vi "MB Serial Receive.vi"(7 "Serial Parameters":T1 {"Slave Address" format="%.0x"}, 8 "error in (no error)":errorcluster, 9 "Timeout":u32=10000, 11 "VISA resource name":refnum<visa-resource-name>) -> (0 "error out":errorcluster, 1 "Exception Code":u8 format="%.0x", 2 "Modbus Data Unit":T2={"Function Code"=1, "Data"=[]} {"Function Code" items=["Read Coils"=1, "Read Discrete Inputs"=2, "Read Holding Registers"=3, "Read Input Registers"=4, "Write Single Coil"=5, "Write Single Register"=6, "Read Exception Status"=7, "Write Multiple Coils"=15, "Write Multiple Registers"=16]; "Data" format="%.0x"}, 3 "VISA resource name out":refnum<visa-resource-name>)   [LabVIEW 2019]
uses:
  MB Modbus Data Unit.ctl
panel:
  out "read modbus frame":errorcluster
  out "read slave address":errorcluster
  # "VI Name: MB Serial Receive.vi\nPurpose: Reads a Modbus message.\nReentrant."
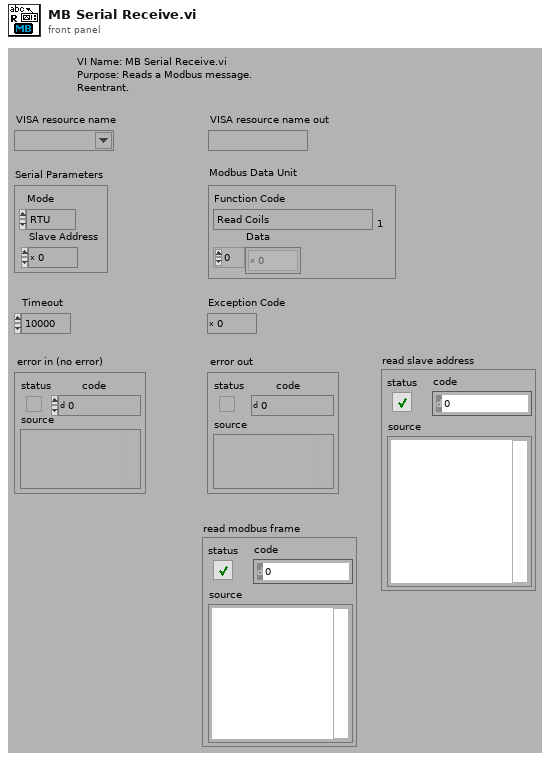
[diagram p1: front panel]
types:
  T1 = cluster{"Mode":enum16{"RTU", "ASCII"}, "Slave Address":u8}
  T2 = typedef "MB Modbus Data Unit.ctl" = cluster{"Function Code":u8, "Data":u8[]}
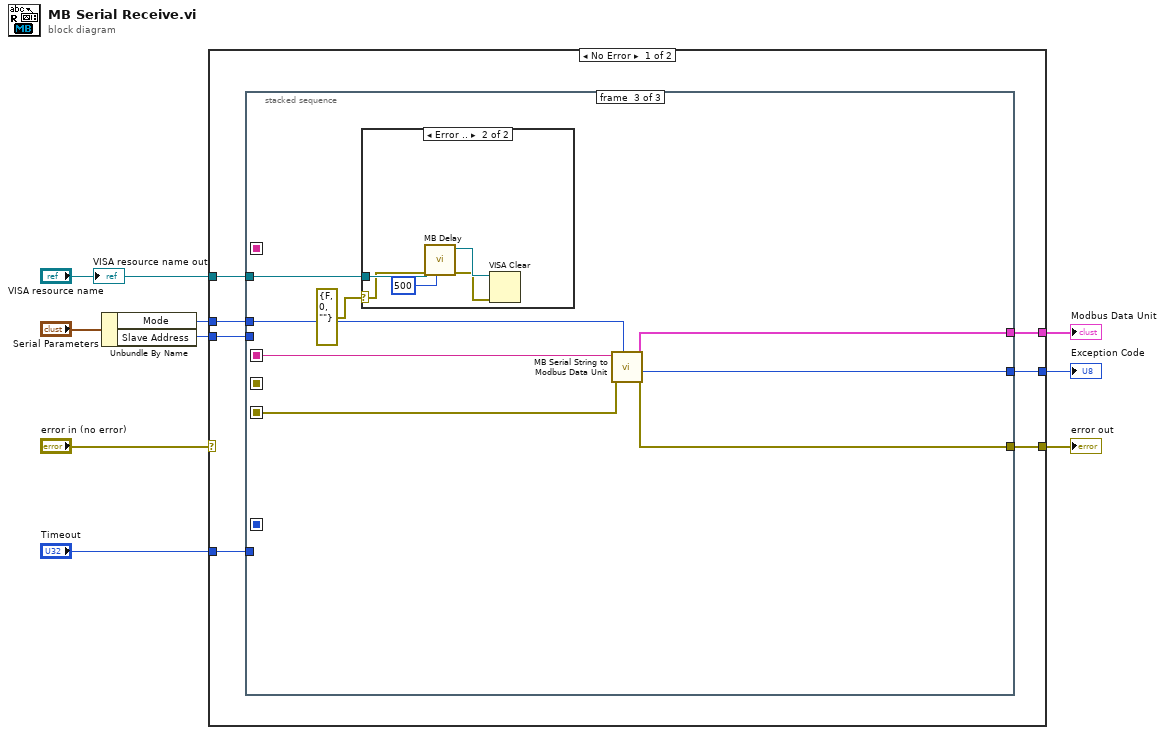
[diagram p0: block diagram]
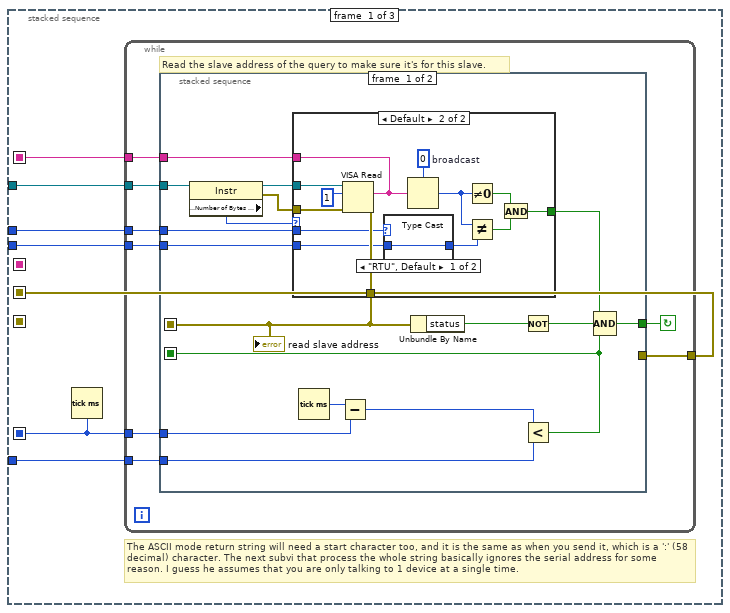
[diagram p2: hidden frame]
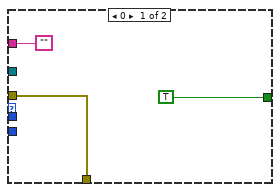
[diagram p3: hidden frame]
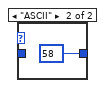
[diagram p4: hidden frame]
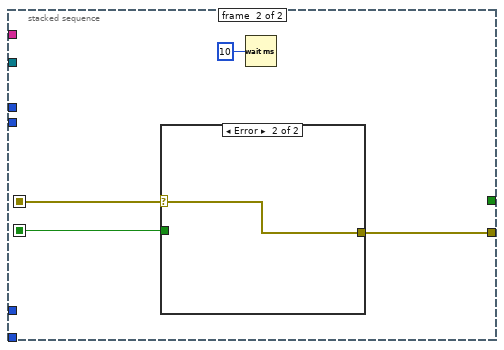
[diagram p5: hidden frame]
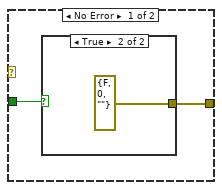
[diagram p6: hidden frame]
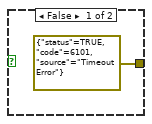
[diagram p7: hidden frame]
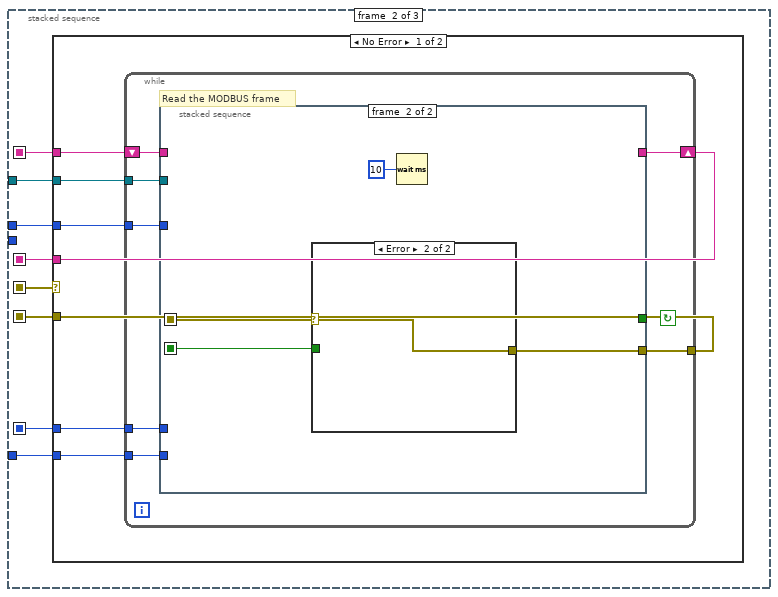
[diagram p8: hidden frame]
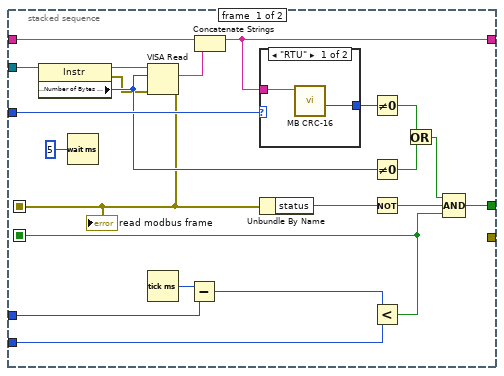
[diagram p9: hidden frame]
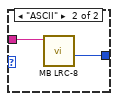
[diagram p10: hidden frame]
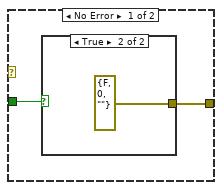
[diagram p11: hidden frame]
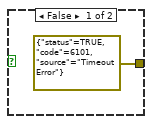
[diagram p12: hidden frame]
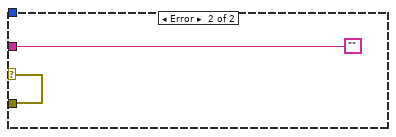
[diagram p13: hidden frame]
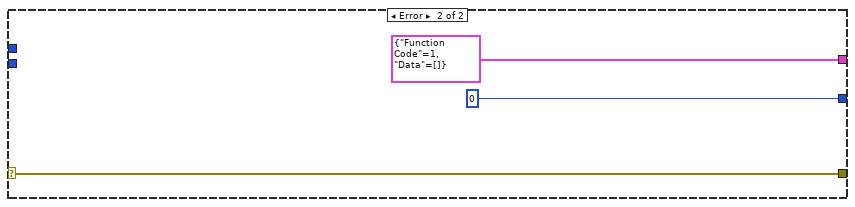
[diagram p15: hidden frame]
diagram:
  n1 = Unbundle By Name("Serial Parameters") -> ("Mode"=w2:enum16{"RTU", "ASCII"}, "Slave Address"=w1:u8)
  n2 = case shown="No Error" "error in (no error)" {
    selector: "error in (no error)" -> [_ w151]
    tunnel: "VISA resource name" -> [w16 _]
    tunnel: w2 -> [w15 _]
    tunnel: [w14 w151] -> w8
    tunnel: [w13 u8 0 ("Exception Code")] -> w6
    tunnel: [w12 T2 {"Function Code"=1, "Data"=[]} ("MODBUS Data Unit")] -> w5
    tunnel: "Timeout" -> [w11 _]
    tunnel: w1 -> [w10 _]
    frame No Error {
      n3 = stacked-sequence {
        seq-local: [_ w81 _] -> [_ _ w141]
        seq-local: [w22 _ _] -> [_ w77 _]
        seq-local: [w20 _ _] -> [_ w79 _]
        seq-local: [_ w78 _] -> [_ _ w138]
        seq-local: [w19 _ _] -> [_ w76 _]
        tunnel: w16 -> [w23 w83 w137]
        tunnel: w15 -> [w17 w82 w143]
        tunnel: [_ _ w142] -> w14
        tunnel: [_ _ w140] -> w13
        tunnel: [_ _ w139] -> w12
        tunnel: w11 -> [w21 w80 _]
        tunnel: w10 -> [w18 _ _]
        frame #0 {
          # "The ASCII mode return string will need a start character too, and it is the same as when you send it, which is a ':' (58 decimal) character. The next subvi that process the whole string basically ignores the serial address for some reason. I guess he assumes that you are only talking to 1 device at a single time."
          n4 = Tick Count (ms)() -> (millisecond timer value=w19:u32)
          n5 = while {
            tunnel: w23 -> [w30]
            tunnel: [w29] -> w22
            tunnel: w21 -> [w28]
            tunnel: [w27] -> w20
            tunnel: w19 -> [w26]
            tunnel: w18 -> [w25]
            tunnel: w17 -> [w24]
            stop <- w31 continue-if-true
            # "Read the slave address of the query to make sure it's for this slave."
            n6 = stacked-sequence {
              seq-local: [w41 _] -> [_ w69]
              seq-local: [w40 _] -> [_ w68]
              tunnel: [w48 _] -> w31
              tunnel: w26 -> [w47 _]
              tunnel: w30 -> [w46 _]
              tunnel: [_ w67] -> w29
              tunnel: w28 -> [w39 _]
              tunnel: [w38 _] -> w27
              tunnel: w25 -> [w33 _]
              tunnel: w24 -> [w32 _]
              frame #0 {
                n7 = property class="Instr"(reference=w46) -> (reference out=w45:refnum<visa-resource-name>, error out=w44:errorcluster, "Serial Settings:Number of Bytes at Serial Port"=w37:u32)  [unwired: 1 in]
                n8 = case shown="Default" w37 {
                  tunnel: w45 -> [_ w64]
                  tunnel: w44 -> [w50 w63]
                  tunnel: [w50 w62] -> w41
                  tunnel: ["" w60] -> w38
                  tunnel: [TRUE w55] -> w36
                  tunnel: w33 -> [_ w54]
                  tunnel: w32 -> [_ w52]
                  frame 0 {
                  }
                  frame Default {
                    w59 = u8 0  # broadcast
                    n9 = VISA Read(VISA resource name=w64, byte count=u32 1, error in (no error)=w63) -> (read buffer=w60:string, error out=w62:errorcluster)  [unwired: 2 out]
                    n10 = case shown="\"RTU\", Default" w52 {
                      tunnel: w54 -> [w65 _]
                      tunnel: [w65 u8 58 ("Slave Address")] -> w53
                      frame "RTU", Default {
                      }
                      frame "ASCII" {
                      }
                    }
                    n11 = Type Cast(type=w59, x=w60) -> (*(type *) &x=w58:u8)
                    n12 = Not Equal To 0?(x=w58) -> (x != 0?=w57:bool)
                    n13 = Not Equal?(x=w58, y=w53) -> (x != y?=w56:bool)
                    n14 = And(x=w57, y=w56) -> (x .and. y?=w55:bool)
                  }
                }
                "read slave address" <- w41
                n15 = Tick Count (ms)() -> (millisecond timer value=w35:u32)
                n16 = Subtract(x=w35, y=w47) -> (x-y=w34:u32)
                n17 = Unbundle By Name(w41) -> ("status"=w43:bool)
                n18 = Not(x=w43) -> (.not. x?=w42:bool)
                n19 = Less?(x=w34, y=w39) -> (x < y?=w40:bool)
                n20 = Compound Arithmetic op=AND(w36, w42, w40) -> (w48:bool)
              }
              frame #1 {
                n21 = case shown="Error" w69 {
                  selector: w69 -> [_ w75]
                  tunnel: w68 -> [w72 _]
                  tunnel: [w71 w75] -> w67
                  frame No Error {
                    n22 = case shown="True" w72 {
                      tunnel: [errorcluster {"status"=TRUE, "code"=6101, "source"="Timeout Error"} ("error out") errorcluster {"status"=FALSE, "code"=0, "source"=""} ("error out")] -> w71
                      frame False {
                      }
                      frame True {
                      }
                    }
                  }
                  frame Error {
                  }
                }
                n23 = Wait (ms)(milliseconds to wait=u32 10) -> ()  [unwired: 1 out]
              }
            }
          }
        }
        frame #1 {
          n24 = case shown="No Error" w77 {
            selector: w77 -> [_ w135]
            tunnel: w83 -> [w90 _]
            tunnel: w82 -> [w89 _]
            tunnel: [w88 ""] -> w81
            tunnel: w80 -> [w87 _]
            tunnel: w79 -> [w86 _]
            tunnel: [w85 w135] -> w78
            tunnel: w76 -> [w84 _]
            frame No Error {
              n25 = while {
                tunnel: w89 -> [w97]
                shift-left: w86 -> [w95]
                shift-right: [w92] -> w88
                tunnel: w90 -> [w96]
                tunnel: [w94] -> w85
                tunnel: w87 -> [w93]
                tunnel: w84 -> [w91]
                stop <- w98 continue-if-true
                # "Read the MODBUS frame"
                n26 = stacked-sequence {
                  seq-local: [w103 _] -> [_ w127]
                  seq-local: [w102 _] -> [_ w126]
                  tunnel: [w119 _] -> w98
                  tunnel: w91 -> [w118 _]
                  tunnel: w97 -> [w117 _]
                  tunnel: w96 -> [w112 _]
                  tunnel: w95 -> [w108 _]
                  tunnel: [w106 _] -> w92
                  tunnel: [_ w125] -> w94
                  tunnel: w93 -> [w101 _]
                  frame #0 {
                    n27 = property class="Instr"(reference=w112) -> (reference out=w111:refnum<visa-resource-name>, error out=w109:errorcluster, "Serial Settings:Number of Bytes at Serial Port"=w110:u32)  [unwired: 1 in]
                    n28 = Wait (ms)(milliseconds to wait=u32 5) -> ()  [unwired: 1 out]
                    n29 = VISA Read(VISA resource name=w111, byte count=w110, error in (no error)=w109) -> (read buffer=w107:string, error out=w103:errorcluster)  [unwired: 2 out]
                    "read modbus frame" <- w103
                    n30 = Tick Count (ms)() -> (millisecond timer value=w120:u32)
                    n31 = Subtract(x=w120, y=w118) -> (x-y=w100:u32)
                    n32 = Concatenate Strings(w108, w107) -> (w106:string)
                    n33 = case shown="\"RTU\"" w117 {
                      tunnel: w106 -> [w122 w124]
                      tunnel: [w121 w123] -> w116
                      frame "RTU" {
                        n34 = call "MB CRC-16.vi"("String"=w122) -> ("CRC-16"=w121:u8)  [unwired: 10 out]
                      }
                      frame "ASCII" {
                        n35 = call "MB LRC-8.vi"("String"=w124) -> ("LRC-8"=w123:u8)  [unwired: 10 out]
                      }
                    }
                    n36 = Unbundle By Name(w103) -> ("status"=w105:bool)
                    n37 = Not Equal To 0?(x=w116) -> (x != 0?=w115:bool)
                    n38 = Not Equal To 0?(x=w110) -> (x != 0?=w113:bool)
                    n39 = Not(x=w105) -> (.not. x?=w104:bool)
                    n40 = Less?(x=w100, y=w101) -> (x < y?=w102:bool)
                    n41 = Or(x=w115, y=w113) -> (x .or. y?=w114:bool)
                    n42 = Compound Arithmetic op=AND(w114, w104, w102) -> (w119:bool)
                  }
                  frame #1 {
                    n43 = case shown="Error" w127 {
                      selector: w127 -> [_ w133]
                      tunnel: w126 -> [w130 _]
                      tunnel: [w129 w133] -> w125
                      frame No Error {
                        n44 = case shown="True" w130 {
                          tunnel: [errorcluster {"status"=TRUE, "code"=6101, "source"="Timeout Error"} ("error out") errorcluster {"status"=FALSE, "code"=0, "source"=""} ("error out")] -> w129
                          frame False {
                          }
                          frame True {
                          }
                        }
                      }
                      frame Error {
                      }
                    }
                    n45 = Wait (ms)(milliseconds to wait=u32 10) -> ()  [unwired: 1 out]
                  }
                }
              }
            }
            frame Error {
            }
          }
        }
        frame #2 {
          n46 = case shown="Error .." errorcluster {"status"=FALSE, "code"=0, "source"=""} ("error IO") {
            selector: errorcluster {"status"=FALSE, "code"=0, "source"=""} ("error IO") -> [_ w145]
            tunnel: w137 -> [_ w148]
            frame No Error {
            }
            frame Error {
              n47 = call "MB Delay.vi"("milliseconds to wait"=u32 500, "error in (no error)"=w145, "VISA Refnum in"=w148) -> ("error out"=w146:errorcluster, "VISA Refnum out"=w147:refnum<visa-resource-name>)  [unwired: 7 in]
              n48 = VISA Clear(VISA resource name=w147, error in (no error)=w146) -> ()  [unwired: 2 out]
            }
          }
          n49 = call "MB Serial String to Modbus Data Unit.vi"("Mode"=w143, "error in (no error)"=w138, "String"=w141) -> ("error out"=w142:errorcluster, "Exception Code"=w140:u8, "Modbus Data Unit"=w139:T2)  [unwired: 1 in, 5 out]
        }
      }
    }
    frame Error {
    }
  }
  "error out" <- w8
  "Exception Code" <- w6
  "Modbus Data Unit" <- w5
  "VISA resource name out" <- "VISA resource name"
